vi "Set_RAW_Array.vi"(0 "reference in":refnum<class "Sig_AI.lvclass">, 5 "RAW":dbl[](array[numeric]), 11 "error in (no error)":errorcluster) -> (4 "reference out":refnum<class "Sig_AI.lvclass">, 15 "error out":errorcluster)   [LabVIEW 2019, in "Sig_AI.lvclass"]
uses:
  Sig_AI.lvclass
  Sig_AI.lvclass/Sig_AI.ctl
  AnalogComparator_class/AnalogComparator.lvclass/AnalogComparator.ctl
  HandleRanges.vi
  HandleAlarms.vi
  subvis/Scale_Raw_to_EU.vi
  AnalogComparator_class/SetValue.vi
  <vilib>/ptbypt/Filters.llb/IIR Filter with I.C. PtByPt.vi
  <vilib>/Utility/error.llb/Error Cluster From Error Code.vi
  AnalogComparator_class/HandleDb.vi
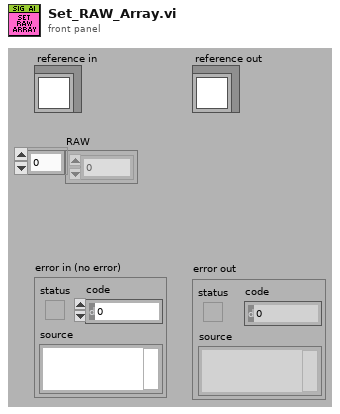
[diagram p1: front panel]
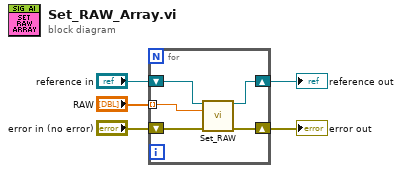
[diagram p0: block diagram]
diagram:
  n1 = for {
    shift-right: [w9] -> w4
    shift-left: "reference in" -> [w10]
    shift-right: [w7] -> w2
    shift-left: "error in (no error)" -> [w8]
    tunnel: "RAW" -> [w6] mode=indexing
    n2 = call "Set_RAW.vi"("reference in"=w10, "RAW"=w6, "error in (no error)"=w8) -> ("reference out"=w9:refnum<class "Sig_AI.lvclass">, "error out"=w7:errorcluster)  [unwired: 11 in]
  }
  "error out" <- w2
  "reference out" <- w4
